vi "Read HDI Slot.vi"(8 "error in":errorcluster, 10 "HDI Slot Number":i32, 11 "WorkTable in":refnum<class "WorkTable Class.lvclass">) -> (0 "error out":errorcluster, 2 "HDI Slot":T1, 3 "WorkTable out":refnum<class "WorkTable Class.lvclass">)   [LabVIEW 2011, in "WorkTable Class.lvclass"]
uses:
  WorkTable Class.lvclass
  Type Definitions/Worktable_HDI Slot.ctl
  Vec3d Class/Vec3d Class.lvclass
  Orient3d Class/Orient3d Class.lvclass
  Utils/Type Definitions/Position_Orientation.ctl
  WorkTable Class.lvclass/WorkTable Class.ctl
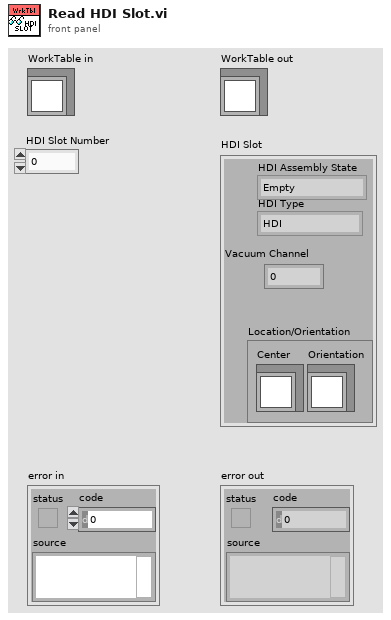
[diagram p1: front panel]
types:
  T1 = typedef "Worktable_HDI Slot.ctl" = cluster{"HDI Assembly State":enum16{"Empty", "Populated"}, "HDI Type":enum16{"HDI", "Polyimide"}, "Vacuum Channel":u32, "Location/Orientation":T2}
  T2 = typedef "Position_Orientation.ctl" = cluster{"Center":refnum<class "Vec3d Class.lvclass">, "Orientation":refnum<class "Orient3d Class.lvclass">}
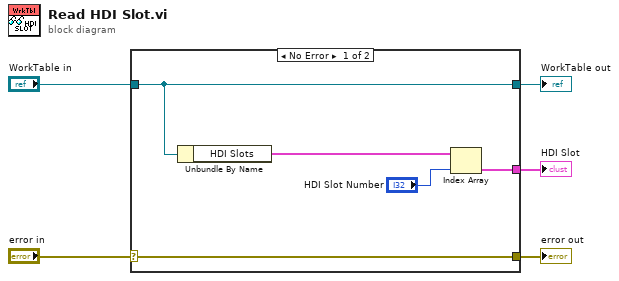
[diagram p0: block diagram]
diagram:
  n1 = case shown="No Error" "error in" {
    selector: "error in" -> [w10 w11]
    tunnel: [w10 w11] -> w4
    tunnel: [w9 w12] -> w2
    tunnel: "WorkTable in" -> [w9 w12]
    tunnel: [w7 _] -> w1
    frame No Error {
      n2 = Unbundle By Name(w9) -> ("HDI Slots"=w8:T1[])
      n3 = Index Array(array=w8, index="HDI Slot Number") -> (element=w7:T1)
    }
    frame Error {
    }
  }
  "error out" <- w4
  "WorkTable out" <- w2
  "HDI Slot" <- w1
